vi "auto avance ralentir.vi"(9 "vitesse gauche":dbl, 10 "temps":dbl, 11 "temps de changement de direction":dbl) -> ()   [LabVIEW 2015]
uses:
  <vilib>/Rock Robotics/WPI/Solenoid/WPI_SolenoidValue.ctl
  <vilib>/Rock Robotics/WPI/Solenoid/WPI_SolenoidSetEnum.vi
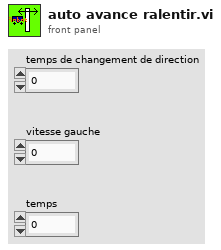
[diagram p1: front panel]
types:
  T1 = typedef "WPI_SolenoidValue.ctl" = enum16{"Off", "On", "Forward", "Reverse"}
  T2 = typedef "WPI_SolenoidDevRef.ctl" = cluster{"DevStatus":errorcluster, "Pneumatics Control Module":u8, "Forward Solenoid Channel":T3, "Reverse Solenoid Channel":T3}
  T3 = typedef "WPI_SolenoidChannel.ctl" = enum8{"Solenoid 0", "Solenoid 1", "Solenoid 2", "Solenoid 3", "Solenoid 4", "Solenoid 5", "Solenoid 6", "Solenoid 7", "Invalid"}
  T4 = typedef "WPI_EncoderDevRef.ctl" = cluster{"DevStatus":errorcluster, "EncoderIndex":T5, "CounterIndex":T6, "DistancePerCount":dbl, "Decoding Type":T7}
  T5 = typedef "FPGA_EncoderIdx.ctl" = enum8{"Enc 0", "Enc 1", "Enc 2", "Enc 3", "Enc 4", "Enc 5", "Enc 6", "Enc 7", "Invalid"}
  T6 = typedef "FPGA_CounterCtrSystemIndex.ctl" = enum8{"Ctr 0", "Ctr 1", "Ctr 2", "Ctr 3", "Ctr 4", "Ctr 5", "Ctr 6", "Ctr 7", "Invalid"}
  T7 = typedef "WPI_EncoderType.ctl" = enum16{"1x", "2x", "4x"}
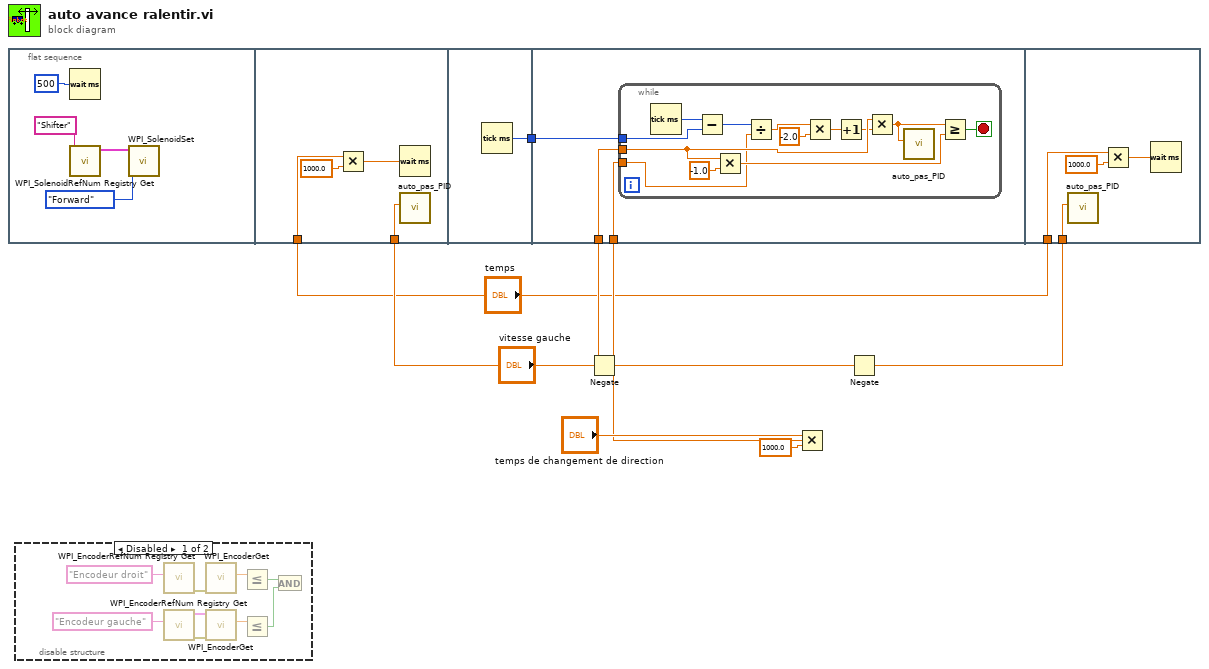
[diagram p0: block diagram]
diagram:
  n1 = flat-sequence {
    tunnel: w3 -> [w16]
    tunnel: "temps" -> [w14]
    tunnel: [w17] -> w8
    tunnel: w8 -> [w20]
    tunnel: w3 -> [w19]
    tunnel: w5 -> [w18]
    tunnel: w2 -> [w37]
    tunnel: "temps" -> [w34]
    frame #0 {
      n2 = Wait (ms)(milliseconds to wait=u32 500) -> ()  [unwired: 1 out]
      n3 = call <vilib>:"WPI_SolenoidRefNum Registry Get.vi"("refnum name"="Shifter") -> ("SolenoidDevRef"=w11:T2)  [unwired: 9 in, 1 out]
      n4 = call-poly <vilib>:"WPI_SolenoidSet.vi"("Value"=WPI_SolenoidValue."Forward", "SolenoidDevRef"=w11) -> ()  [unwired: 8 in, 2 out]
    }
    frame #1 {
      n5 = Multiply(x=w14, y=1000.0) -> (x*y=w13:dbl)
      n6 = Wait (ms)(milliseconds to wait=w13) -> ()  [unwired: 1 out]
      n7 = call "auto_pas_PID.vi"("vitesse voulu"=w16) -> ()  [unwired: 11 in]
    }
    frame #2 {
      n8 = Tick Count (ms)() -> (millisecond timer value=w17:u32)
    }
    frame #3 {
      n9 = while {
        tunnel: w20 -> [w24]
        tunnel: w19 -> [w32]
        tunnel: w18 -> [w30]
        stop <- w21 stop-if-true
        n10 = Tick Count (ms)() -> (millisecond timer value=w23:u32)
        n11 = Subtract(x=w23, y=w24) -> (x-y=w29:u32)
        n12 = Multiply(x=w32, y=-1.0) -> (x*y=w31:dbl)
        n13 = Divide(x=w29, y=w30) -> (x/y=w27:dbl)
        n14 = Multiply(x=w27, y=-2.0) -> (x*y=w26:dbl)
        n15 = Increment(x=w26) -> (x+1=w25:dbl)
        n16 = Multiply(x=w32, y=w25) -> (x*y=w22:dbl)
        n17 = call "auto_pas_PID.vi"("vitesse voulu"=w22) -> ()  [unwired: 11 in]
        n18 = Greater Or Equal?(x=w22, y=w31) -> (x >= y?=w21:bool)
      }
    }
    frame #4 {
      n19 = call "auto_pas_PID.vi"("vitesse voulu"=w37) -> ()  [unwired: 11 in]
      n20 = Multiply(x=w34, y=1000.0) -> (x*y=w36:dbl)
      n21 = Wait (ms)(milliseconds to wait=w36) -> ()  [unwired: 1 out]
    }
  }
  n22 = disable-structure shown="Disabled" {
    frame Disabled {
      n23 = call <vilib>:"WPI_EncoderRefNum Registry Get.vi"("refnum name"="Encodeur droit") -> ("error out"=w38:errorcluster)  [unwired: 9 in, 1 out]
      n24 = call <vilib>:"WPI_EncoderRefNum Registry Get.vi"("refnum name"="Encodeur gauche") -> ("error out"=w40:errorcluster, "EncoderDevRef"=w41:T4)  [unwired: 9 in]
      n25 = call <vilib>:"WPI_EncoderGet.vi"("error in (no error)"=w38) -> ("Distance"=w43:dbl)  [unwired: 5 in, 5 out]
      n26 = call <vilib>:"WPI_EncoderGet.vi"("error in (no error)"=w40, "EncoderDevRef"=w41) -> ("Distance"=w46:dbl)  [unwired: 4 in, 5 out]
      n27 = Less Or Equal?(x=w43) -> (x <= y?=w44:bool)  [unwired: 1 in]
      n28 = Less Or Equal?(x=w46) -> (x <= y?=w45:bool)  [unwired: 1 in]
      n29 = And(x=w44, y=w45) -> ()  [unwired: 1 out]
    }
    frame Enabled {
    }
  }
  n30 = Negate(x="vitesse gauche") -> (-x=w3:dbl)
  n31 = Multiply(x="temps de changement de direction", y=1000.0) -> (x*y=w5:dbl)
  n32 = Negate(x=w3) -> (-x=w2:dbl)
